vi "header_dialog.vi"(8 "error in (no error)":errorcluster, 11 "header string in":string) -> (0 "error out":errorcluster)   [LabVIEW 2010, in "XImage.xctl"]
uses:
  XImage.xctl
panel:
  in  "saveButton":bool
  in  "closeButton":bool
  out "XML Header":string
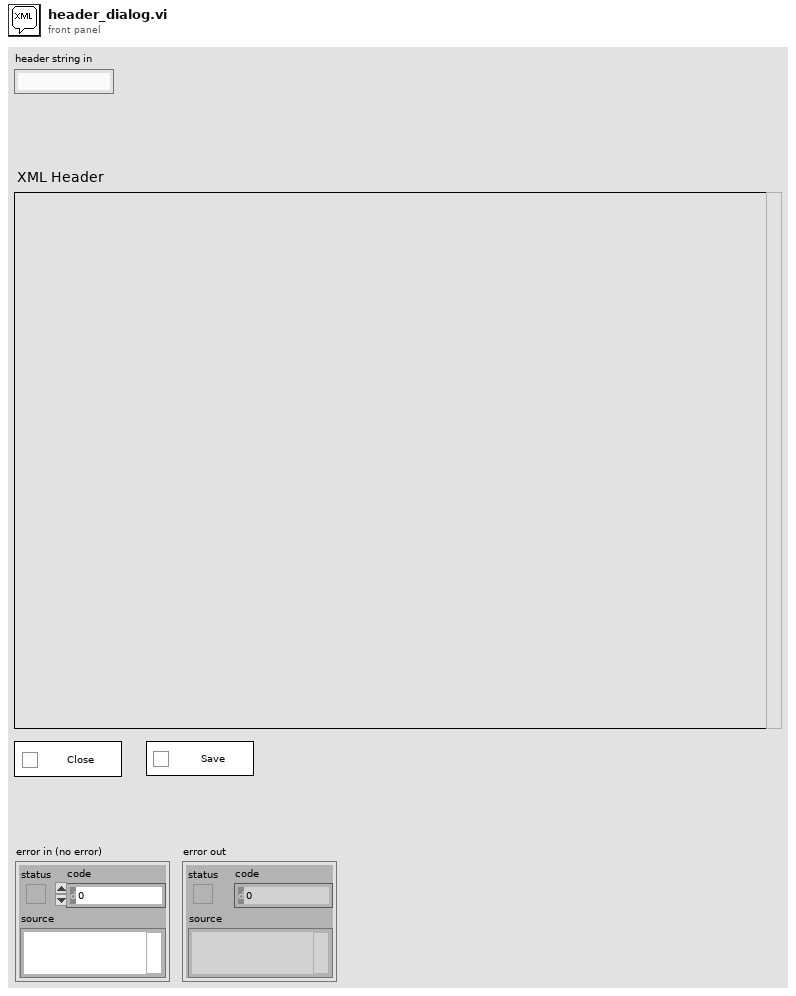
[diagram p1: front panel]
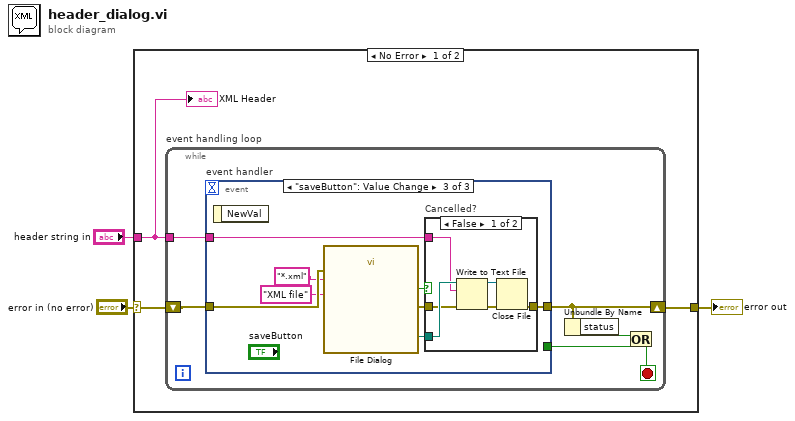
[diagram p0: block diagram]
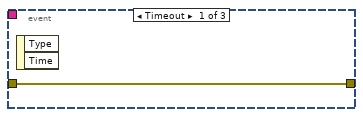
[diagram p2: hidden frame]
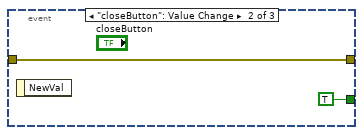
[diagram p3: hidden frame]
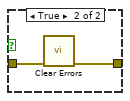
[diagram p4: hidden frame]
diagram:
  n1 = case shown="No Error" "error in (no error)" {
    selector: "error in (no error)" -> [w6 w32]
    tunnel: [w5 w32] -> w2
    tunnel: "header string in" -> [w4 _]
    frame No Error {
      n2 = while "event handling loop" {
        shift-right: [w11] -> w5
        shift-left: w6 -> [w12]
        tunnel: w4 -> [w7]
        stop <- w8 stop-if-true
        n3 = event "event handler" shown="[2] \"saveButton\": Value Change" {
          selector: _ -> [_ _ _]
          dyn-events: _ -> [_ _ _]
          timeout: _ -> [_ _ _]
          tunnel: [w13 w15 w20] -> w11
          tunnel: w12 -> [w13 w15 w23]
          tunnel: [_ TRUE _] -> w9
          tunnel: w7 -> [_ _ w17]
          event Timeout {
            n4 = event-data() -> ()  [unwired: 1 in, 2 out]
          }
          event "closeButton": Value Change {
            n5 = event-data() -> ()  [unwired: 1 in, 1 out]
          }
          event "saveButton": Value Change {
            n6 = event-data() -> ()  [unwired: 1 in, 1 out]
            n7 = call "File Dialog"("error in"=w23, "pattern (all files)"="*.xml", "pattern label"="XML file") -> ("selected path"=w22:path, "cancelled"=w19:bool, "error out"=w21:errorcluster)  [unwired: 9 in, 1 out]
            n8 = case "Cancelled?" shown="False" w19 {
              tunnel: w22 -> [w29 _]
              tunnel: w21 -> [w28 w31]
              tunnel: [w25 w30] -> w20
              tunnel: w17 -> [w24 _]
              frame False {
                n9 = Write to Text File(file (use dialog)=w29, text=w24, error in=w28) -> (refnum out=w27:refnum<file>, error out=w26:errorcluster)  [unwired: 1 in, 1 out]
                n10 = Close File(refnum=w27, error in=w26) -> (error out=w25:errorcluster)  [unwired: 1 out]
              }
              frame True {
                n11 = call <vilib>:"Clear Errors.vi"("error in (no error)"=w31) -> ("error out"=w30:errorcluster)  [unwired: 6 in]
              }
            }
          }
        }
        n12 = Unbundle By Name(w11) -> ("status"=w10:bool)
        n13 = Or(x=w10, y=w9) -> (x .or. y?=w8:bool)
      }
      "XML Header" <- w4
    }
    frame Error {
    }
  }
  "error out" <- w2
